vi "Connect.vi"(8 "error in (no error)":errorcluster, 9 "ConfigDir":string, 10 "nSensorIP":u32, 11 "nHostIP":u32) -> (0 "error out":errorcluster, 1 "ConfigDir out":string, 3 "function return":i32)   [LabVIEW 2017, in "BonTechWrapperLibrary.lvlib"]
doc: "extern \"C\" BONTECHLIBRARY_API int __stdcall Connect(unsigned int nHostIP, unsigned int nSensorIP, LPTSTR ConfigDir);"
uses:
  BonTechWrapperLibrary.lvlib
  BonTechWrapperLibrary.dll
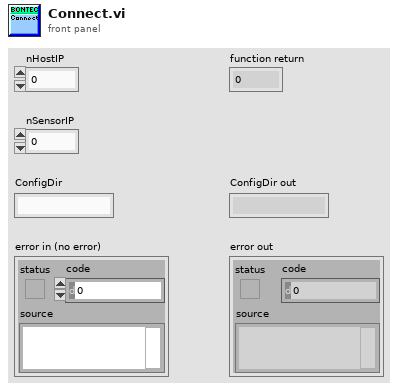
[diagram p1: front panel]
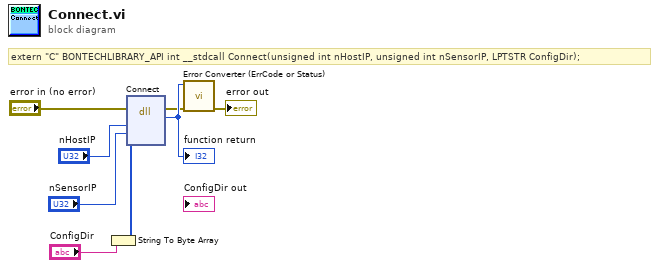
[diagram p0: block diagram]
diagram:
  # "extern \"C\" BONTECHLIBRARY_API int __stdcall Connect(unsigned int nHostIP, unsigned int nSensorIP, LPTSTR ConfigDir);"
  n1 = String To Byte Array(string="ConfigDir") -> (unsigned byte array=w1:u8[])
  n2 = dll-call lib="C:/Users/Achuthaperumal/SourceCodes/BonTechWrapperLibrary/BonTechWrapperLibrary/x64/Release/BonTechWrapperLibrary.*" fn="Connect"(error in="error in (no error)", "nHostIP"="nHostIP", "nSensorIP"="nSensorIP", "ConfigDir"=w1) -> (error out=w3:errorcluster, "return type"=w8:i32)  [unwired: 5 in, 1 out]
  "function return" <- w8
  n3 = call "Error Converter (ErrCode or Status).vi"("error in (no error)"=w3, "error code"=w8) -> ("error out"=→"error out":errorcluster)  [unwired: 9 in]
